vi "Render Template.vi"(8 "error in (no error)":errorcluster, 10 "Template":string, 11 "BasicTemplater in":refnum<class "BasicTemplater.lvclass">) -> (0 "error out":errorcluster, 2 "Output":string, 3 "BasicTemplater out":refnum<class "BasicTemplater.lvclass">)   [LabVIEW 2020, in "HTTP Server.lvlib" / "BasicTemplater.lvclass"]
uses:
  BasicTemplater.lvclass
  BasicTemplater.lvclass/BasicTemplater.ctl
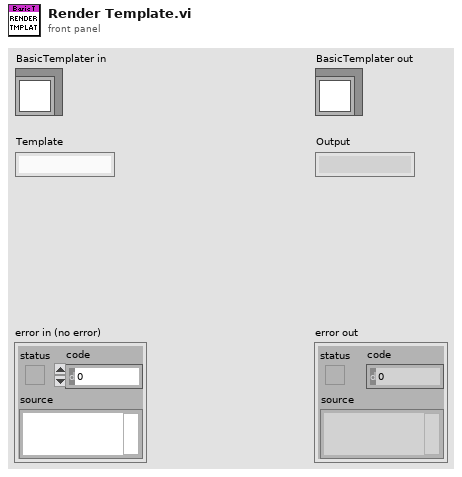
[diagram p1: front panel]
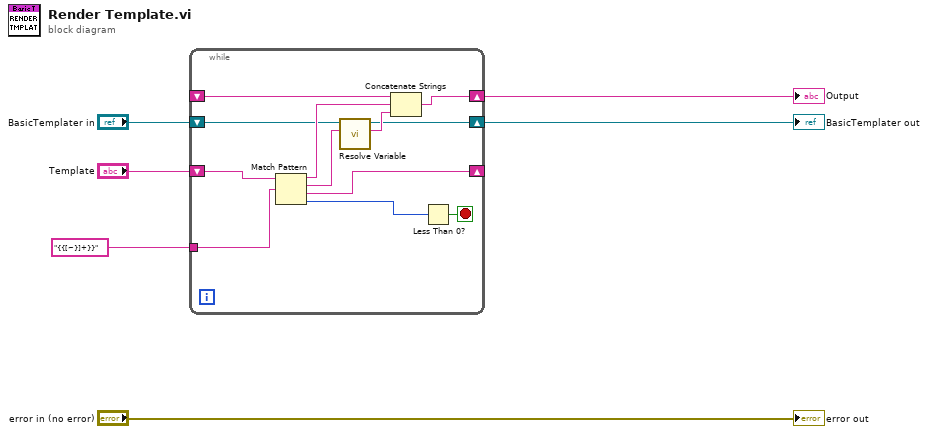
[diagram p0: block diagram]
diagram:
  n1 = while {
    shift-right: [w14] -> w1
    shift-left: _ -> [w16]
    tunnel: "{{[~}]+}}" ("regular expression") -> [w12]
    shift-right: [w11] -> _
    shift-left: "Template" -> [w17]
    shift-right: [w7] -> w2
    shift-left: "BasicTemplater in" -> [w13]
    stop <- w18 stop-if-true
    n2 = Match Pattern(string=w17, regular expression=w12) -> (before substring=w15:string, match substring=w10:string, after substring=w11:string, offset past match=w9:i32)  [unwired: 1 in]
    n3 = call "Resolve Variable.vi"("Variable Name"=w10, "BasicTemplater in"=w13) -> ("Value"=w8:string, "BasicTemplater out"=w7:refnum<class "BasicTemplater.lvclass">)  [unwired: 6 in, 2 out]
    n4 = Concatenate Strings(w16, w15, w8) -> (w14:string)
    n5 = Less Than 0?(x=w9) -> (x < 0?=w18:bool)
  }
  "BasicTemplater out" <- w2
  "Output" <- w1
  "error out" <- "error in (no error)"
